vi "dvp Vi Get Ae Target.vi"(10 "pAeTarget":i32, 11 "handle":u32) -> (2 "pAeTarget out":i32, 3 "function return":u32(ring))   [LabVIEW 2018, in "LabViewDVPCamera.lvlib"]
doc: "LabviewDvp2Api dvpStatus dvpViGetAeTarget(dvpHandle handle, dvpInt32 *pAeTarget);"
uses:
  LabViewDVPCamera.lvlib
  LabViewDVPCamera/LabViewDVPCamera.dll
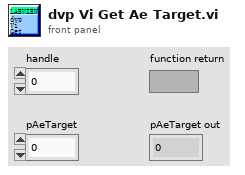
[diagram p1: front panel]
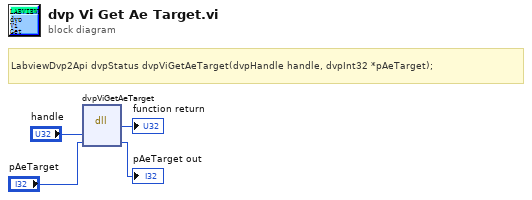
[diagram p0: block diagram]
diagram:
  # "LabviewDvp2Api dvpStatus dvpViGetAeTarget(dvpHandle handle, dvpInt32 *pAeTarget);"
  n1 = dll-call lib="C:/Program Files (x86)/DVP2 Labview cn 64/Sample/LabViewDVPCamera/LabViewDVPCamera.*" fn="dvpViGetAeTarget"("handle"="handle", "pAeTarget"="pAeTarget") -> (→"function return":u32, "pAeTarget"=→"pAeTarget out":i32)  [unwired: 4 in, 2 out]
